vi "Save Linked List.vi"(6 "Persistence":refnum<class "IPersist.lvclass">, 8 "error in (no error)":errorcluster, 9 "File Name":string, 10 "Folder":path, 11 "Linked List Ref":refnum<data-value>) -> (0 "error out":errorcluster, 3 "Linked List Ref out":refnum<data-value>)   [LabVIEW 2020, in "Linked Lists.lvlib" / "Linked List Ref.lvclass"]
uses:
  <vilib>/gpm_packages/@cs/linked-list/Source/Linked List/Linked List Ref/Linked List Ref.lvclass
  <vilib>/gpm_packages/@cs/linked-list/Source/Linked List/ILinkedList/ILinked List.lvclass
  <vilib>/gpm_packages/@cs/persistence/source/IPersist/IPersist.lvclass
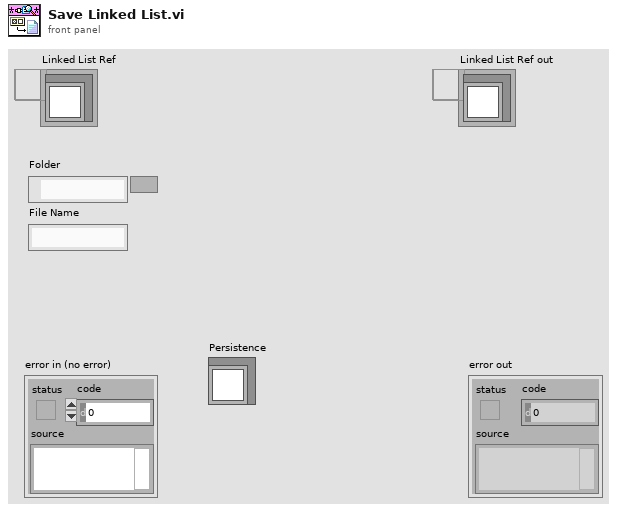
[diagram p1: front panel]
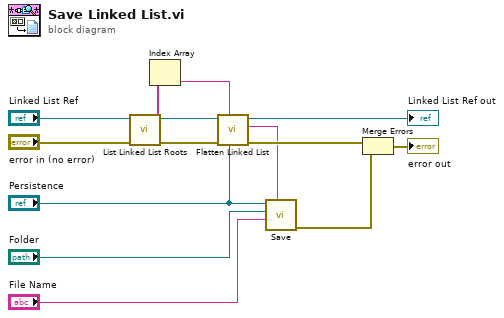
[diagram p0: block diagram]
diagram:
  n1 = call <vilib>:"List Linked List Roots.vi"("error in (no error)"="error in (no error)", "Linked List Ref"="Linked List Ref") -> ("error out"=w7:errorcluster, "Root IDs"=w11:string[], "Linked List Ref out"=w13:refnum<data-value>)  [unwired: 6 in, 1 out]
  n2 = Index Array(array=w11) -> (element=w10:string)  [unwired: 1 in]
  n3 = call <vilib>:"Flatten Linked List.vi"("Persistence"="Persistence", "Linked List ID"=w10, "error in (no error)"=w7, "Linked List Ref"=w13) -> ("error out"=w6:errorcluster, "Flattened Linked List"=w4:string, "Linked List Ref out"=→"Linked List Ref out":refnum<data-value>)  [unwired: 5 in]
  n4 = call-dynamic "Save.vi"("Flattened String"=w4, "File Name"="File Name", "Folder"="Folder", "IPersist in"="Persistence") -> ("error out"=w3:errorcluster)  [unwired: 6 in, 1 out]
  n5 = Merge Errors(w6, w3) -> (→"error out":errorcluster)
